vi "Match Regex.vi"(7 "regular expression":string, 8 "error in (no error)":errorcluster, 9 "offset":i32, 11 "String":string) -> (0 "error out":errorcluster, 1 "offset past match":i32, 2 "submatch 1":string, 3 "whole match":string)   [LabVIEW 2017, in "TOML.lvlib"]
uses:
  TOML.lvlib
  <vilib>/Utility/error.llb/Error Cluster From Error Code.vi
  <vilib>/regexp/Match Regular Expression.xnode
  <vilib>/ErrorRing/Error Ring.xnode
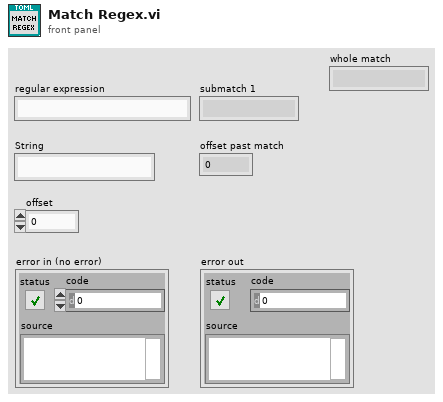
[diagram p1: front panel]
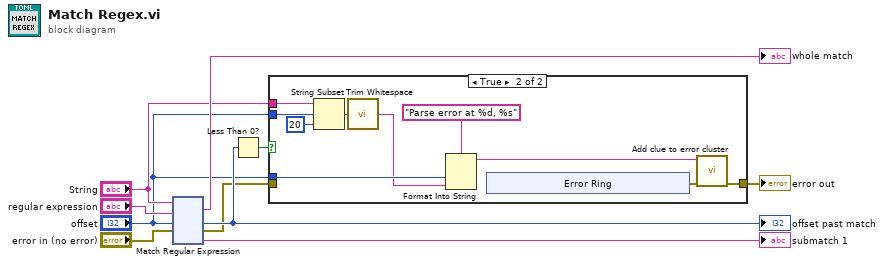
[diagram p0: block diagram]
diagram:
  n1 = xnode "Match Regular Expression"("input string"="String", "regular expression"="regular expression", "offset (0)"="offset", "error in"="error in (no error)") -> ("whole match"=→"whole match":string, "offset past match"=w9:i32, "error out"=w4:errorcluster, "submatch 1"=→"submatch 1":string)  [unwired: 2 in, 2 out]
  "offset past match" <- w9
  n2 = Less Than 0?(x=w9) -> (x < 0?=w5:bool)
  n3 = case shown="True" w5 {
    tunnel: "offset" -> [_ w21]
    tunnel: w4 -> [w11 _]
    tunnel: [w11 w18] -> w3
    tunnel: "String" -> [_ w16]
    tunnel: "offset" -> [_ w15]
    frame False {
    }
    frame True {
      n4 = String Subset(string=w16, offset (0)=w15, length (rest)=20 ("length (rest)")) -> (substring=w13:string)
      n5 = call <vilib>:"Trim Whitespace.vi"("string"=w13) -> ("trimmed string"=w12:string)  [unwired: 1 in]
      n6 = Format Into String(format string="Parse error at %d, %s", w21, w12) -> (resulting string=w17:string)  [unwired: 2 in, 1 out]
      n7 = xnode "Error Ring"() -> ("error out"=w19:errorcluster)
      n8 = call "Add clue to error cluster.vi"("error in (no error)"=w19, "String"=w17) -> ("error out"=w18:errorcluster)  [unwired: 9 in]
    }
  }
  "error out" <- w3
